vi "button press.vi"(11 "button IN":bool=TRUE) -> (3 "Button Pressed?":bool=TRUE)   [LabVIEW 2023]
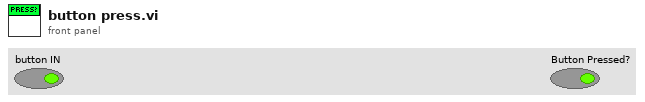
[diagram p1: front panel]
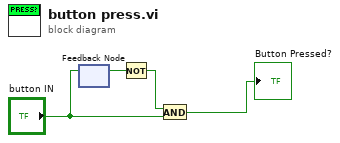
[diagram p0: block diagram]
diagram:
  n1 = feedback-in #1("button IN") -> ()
  n2 = feedback #1() -> (w4:bool)  [unwired: 1 in]
  n3 = Not(x=w4) -> (.not. x?=w2:bool)
  n4 = And(x=w2, y="button IN") -> (x .and. y?=→"Button Pressed?":bool)
